vi "DAQ_finite.vi"(8 "error in":errorcluster) -> (0 "error out":errorcluster, 3 "task out":refnum<k21>)   [LabVIEW 2019]
uses:
  <vilib>/DAQmx/create/channels.llb/DAQmx Create Channel (AI-Voltage-Basic).vi
  <vilib>/DAQmx/configure/timing.llb/DAQmx Timing (Sample Clock).vi
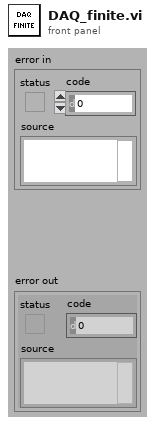
[diagram p1: front panel]
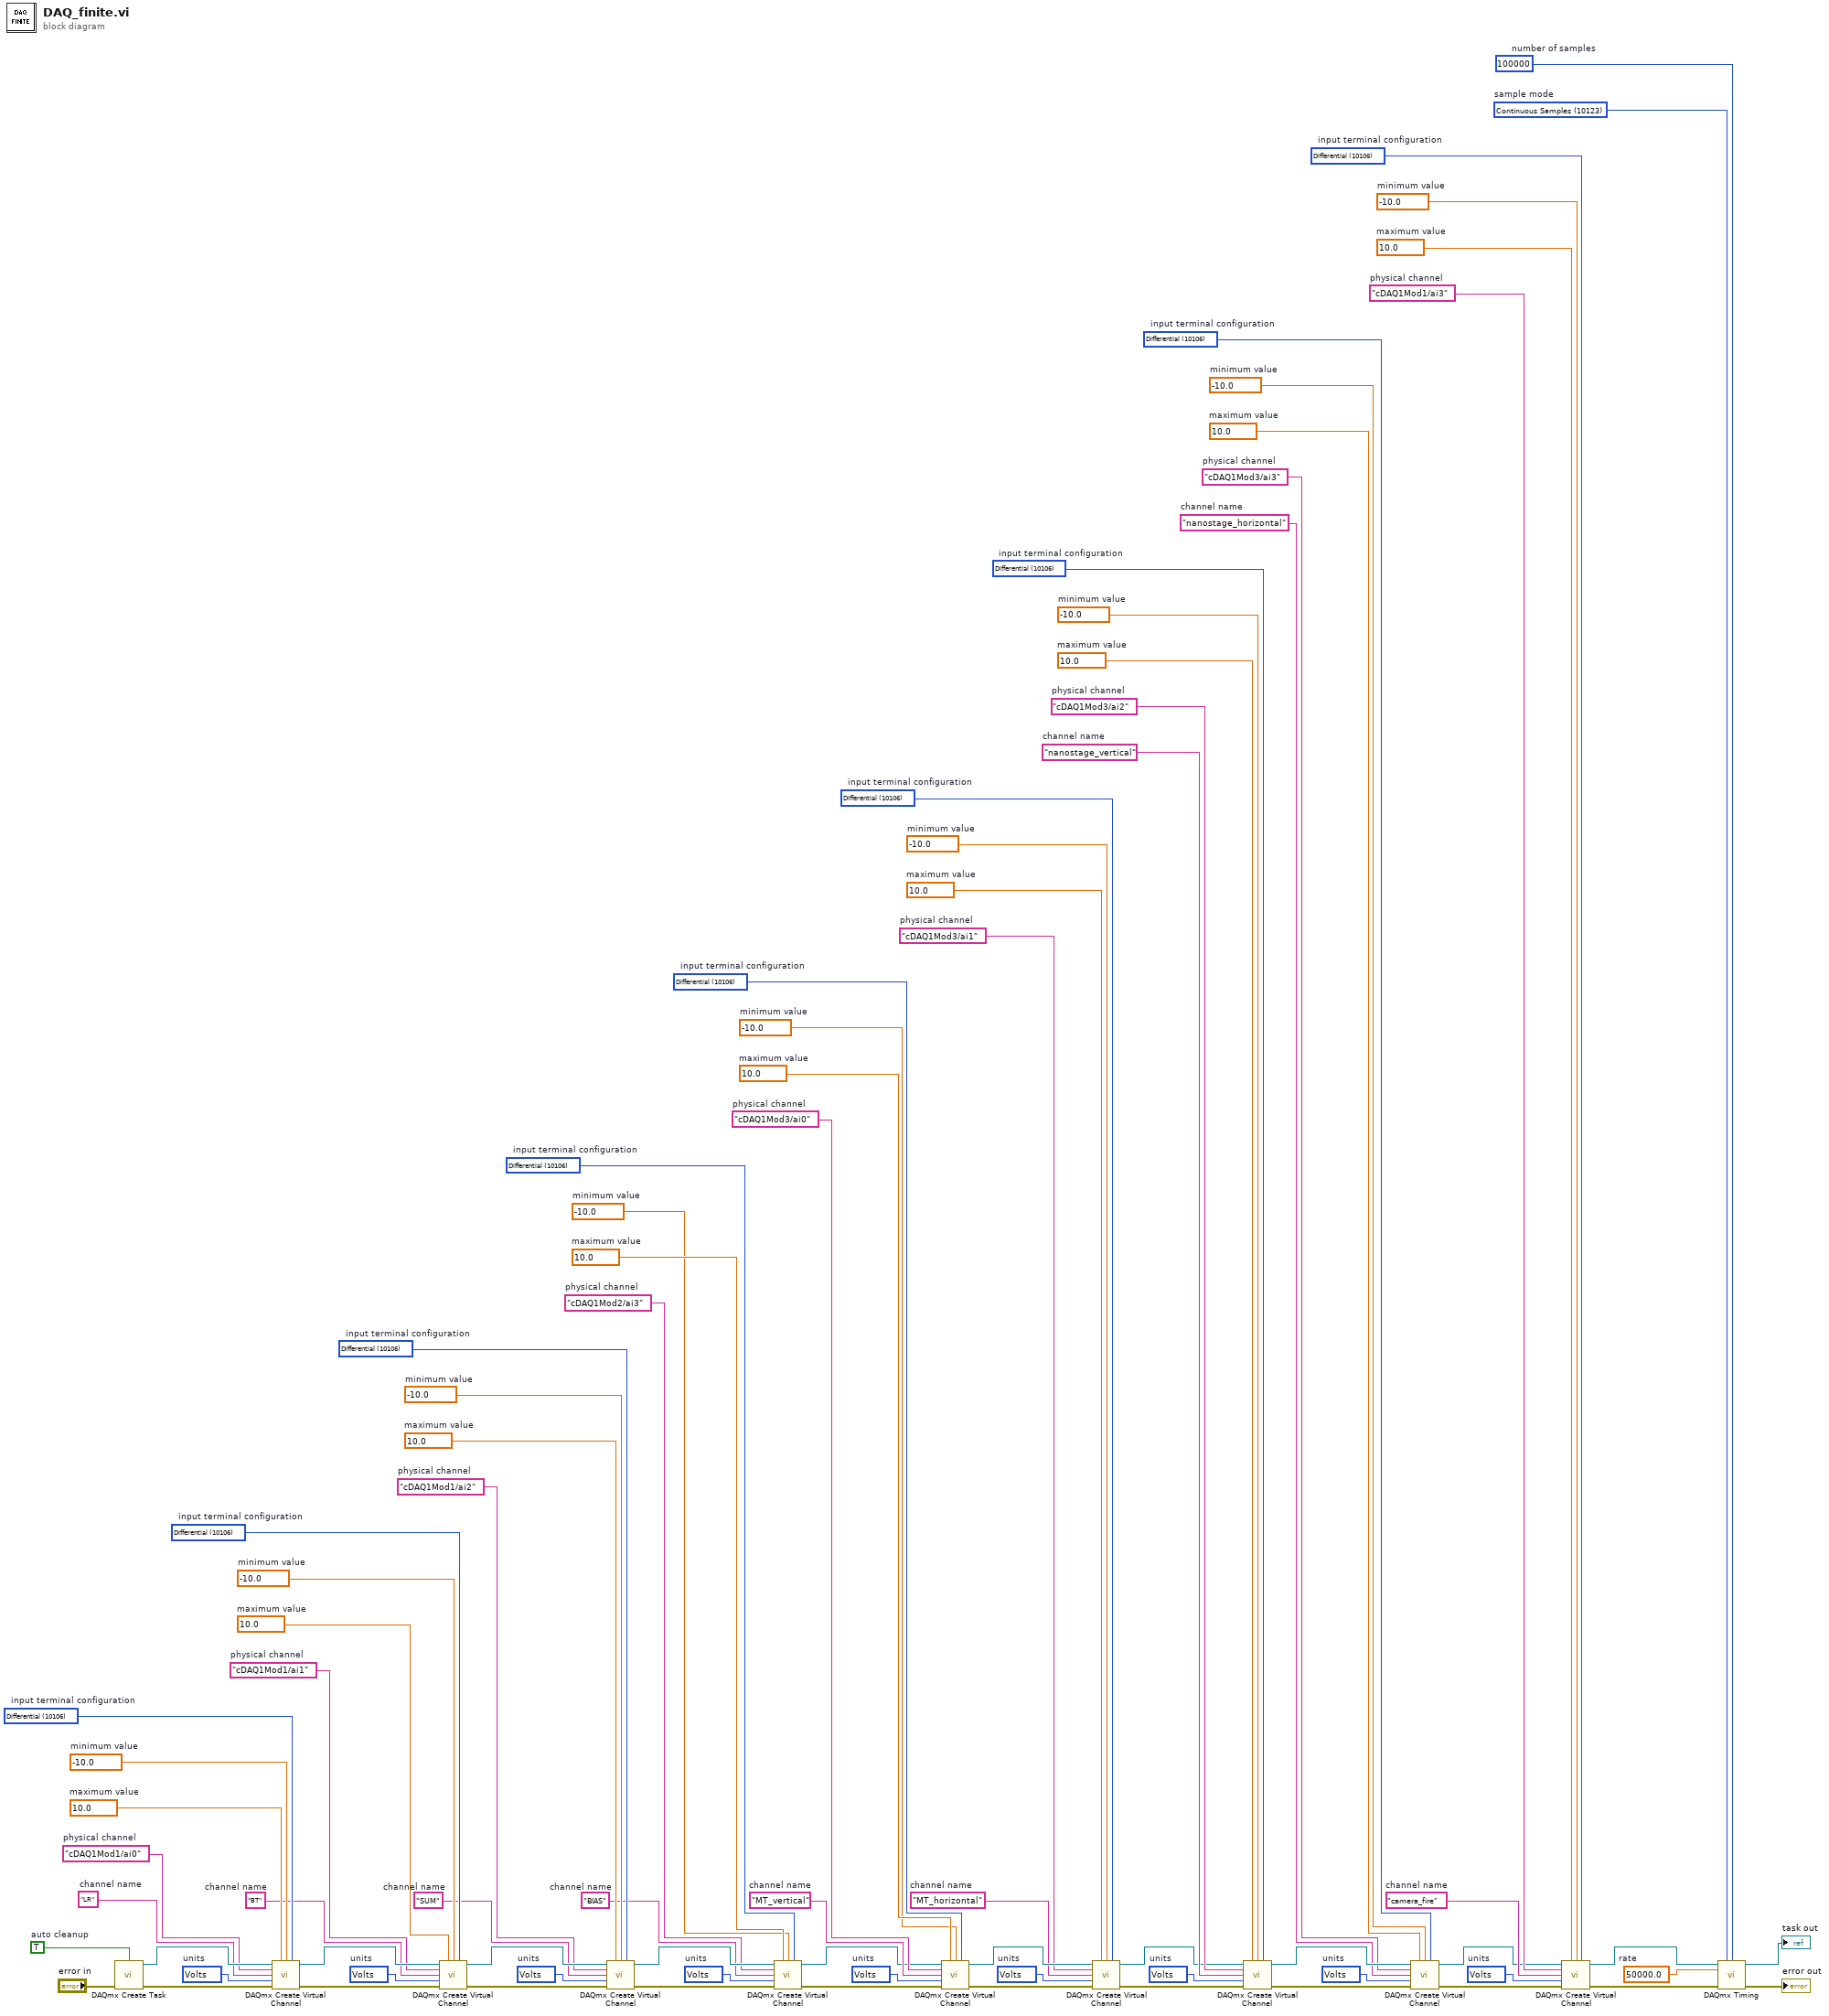
[diagram p0: block diagram]
diagram:
  w3 = 10123 items=["Finite Samples"=10178, "Continuous Samples"=10123, "Hardware Timed Single Point"=12522]  # sample mode
  w4 = 100000  # number of samples
  w5 = 50000.0  # rate
  w10 = 10106 items=["default"=-1, "RSE"=10083, "NRSE"=10078, "Differential"=10106, "Pseudodifferential"=12529]  # input terminal configuration
  w11 = 10348 items=["Volts"=10348, "From Custom Scale"=10065]  # units
  w12 = "camera_fire"  # channel name
  w13 = -10.0  # minimum value
  w14 = 10.0  # maximum value
  w15 = "cDAQ1Mod1/ai3"  # physical channel
  w20 = 10106 items=["default"=-1, "RSE"=10083, "NRSE"=10078, "Differential"=10106, "Pseudodifferential"=12529]  # input terminal configuration
  w21 = 10348 items=["Volts"=10348, "From Custom Scale"=10065]  # units
  w22 = "nanostage_horizontal"  # channel name
  w23 = -10.0  # minimum value
  w24 = 10.0  # maximum value
  w25 = "cDAQ1Mod3/ai3"  # physical channel
  w27 = 10106 items=["default"=-1, "RSE"=10083, "NRSE"=10078, "Differential"=10106, "Pseudodifferential"=12529]  # input terminal configuration
  w28 = 10348 items=["Volts"=10348, "From Custom Scale"=10065]  # units
  w29 = "nanostage_vertical"  # channel name
  w31 = -10.0  # minimum value
  w32 = 10.0  # maximum value
  w33 = "cDAQ1Mod3/ai2"  # physical channel
  w34 = 10106 items=["default"=-1, "RSE"=10083, "NRSE"=10078, "Differential"=10106, "Pseudodifferential"=12529]  # input terminal configuration
  w35 = 10348 items=["Volts"=10348, "From Custom Scale"=10065]  # units
  w36 = "MT_horizontal"  # channel name
  w37 = -10.0  # minimum value
  w38 = 10.0  # maximum value
  w39 = "cDAQ1Mod3/ai1"  # physical channel
  w41 = 10106 items=["default"=-1, "RSE"=10083, "NRSE"=10078, "Differential"=10106, "Pseudodifferential"=12529]  # input terminal configuration
  w42 = 10348 items=["Volts"=10348, "From Custom Scale"=10065]  # units
  w43 = "MT_vertical"  # channel name
  w45 = -10.0  # minimum value
  w46 = 10.0  # maximum value
  w47 = "cDAQ1Mod3/ai0"  # physical channel
  w48 = 10106 items=["default"=-1, "RSE"=10083, "NRSE"=10078, "Differential"=10106, "Pseudodifferential"=12529]  # input terminal configuration
  w49 = 10348 items=["Volts"=10348, "From Custom Scale"=10065]  # units
  w50 = "BIAS"  # channel name
  w51 = -10.0  # minimum value
  w52 = 10.0  # maximum value
  w53 = "cDAQ1Mod2/ai3"  # physical channel
  w55 = 10106 items=["default"=-1, "RSE"=10083, "NRSE"=10078, "Differential"=10106, "Pseudodifferential"=12529]  # input terminal configuration
  w56 = 10348 items=["Volts"=10348, "From Custom Scale"=10065]  # units
  w57 = "SUM"  # channel name
  w59 = -10.0  # minimum value
  w60 = 10.0  # maximum value
  w61 = "cDAQ1Mod1/ai2"  # physical channel
  w63 = 10106 items=["default"=-1, "RSE"=10083, "NRSE"=10078, "Differential"=10106, "Pseudodifferential"=12529]  # input terminal configuration
  w64 = 10348 items=["Volts"=10348, "From Custom Scale"=10065]  # units
  w65 = "BT"  # channel name
  w67 = -10.0  # minimum value
  w68 = 10.0  # maximum value
  w69 = "cDAQ1Mod1/ai1"  # physical channel
  w71 = 10106 items=["default"=-1, "RSE"=10083, "NRSE"=10078, "Differential"=10106, "Pseudodifferential"=12529]  # input terminal configuration
  w72 = 10348 items=["Volts"=10348, "From Custom Scale"=10065]  # units
  w73 = "LR"  # channel name
  w75 = -10.0  # minimum value
  w76 = 10.0  # maximum value
  w77 = "cDAQ1Mod1/ai0"  # physical channel
  w79 = TRUE  # auto cleanup
  n1 = call <vilib>:"DAQmx Create Task.vi"("auto cleanup"=w79, "error in"="error in") -> ("task out"=w78:refnum<k21>, "error out"=w80:errorcluster)  [unwired: 12 in]
  n2 = call-poly <vilib>:"DAQmx Create Virtual Channel.vi"("task in"=w78, "maximum value"=w76, "minimum value"=w75, "input terminal configuration"=w71, "physical channels"=w77, "name to assign"=w73, "units"=w72, "error in"=w80) -> ("task out"=w70:refnum<k21>, "error out"=w74:errorcluster)  [unwired: 6 in]
  n3 = call-poly <vilib>:"DAQmx Create Virtual Channel.vi"("task in"=w70, "maximum value"=w68, "minimum value"=w67, "input terminal configuration"=w63, "physical channels"=w69, "name to assign"=w65, "units"=w64, "error in"=w74) -> ("task out"=w62:refnum<k21>, "error out"=w66:errorcluster)  [unwired: 6 in]
  n4 = call-poly <vilib>:"DAQmx Create Virtual Channel.vi"("task in"=w62, "maximum value"=w60, "minimum value"=w59, "input terminal configuration"=w55, "physical channels"=w61, "name to assign"=w57, "units"=w56, "error in"=w66) -> ("task out"=w54:refnum<k21>, "error out"=w58:errorcluster)  [unwired: 6 in]
  n5 = call-poly <vilib>:"DAQmx Create Virtual Channel.vi"("task in"=w54, "maximum value"=w52, "minimum value"=w51, "input terminal configuration"=w48, "physical channels"=w53, "name to assign"=w50, "units"=w49, "error in"=w58) -> ("task out"=w17:refnum<k21>, "error out"=w16:errorcluster)  [unwired: 6 in]
  n6 = call-poly <vilib>:"DAQmx Create Virtual Channel.vi"("task in"=w17, "maximum value"=w46, "minimum value"=w45, "input terminal configuration"=w41, "physical channels"=w47, "name to assign"=w43, "units"=w42, "error in"=w16) -> ("task out"=w40:refnum<k21>, "error out"=w44:errorcluster)  [unwired: 6 in]
  n7 = call-poly <vilib>:"DAQmx Create Virtual Channel.vi"("task in"=w40, "maximum value"=w38, "minimum value"=w37, "input terminal configuration"=w34, "physical channels"=w39, "name to assign"=w36, "units"=w35, "error in"=w44) -> ("task out"=w19:refnum<k21>, "error out"=w18:errorcluster)  [unwired: 6 in]
  n8 = call-poly <vilib>:"DAQmx Create Virtual Channel.vi"("task in"=w19, "maximum value"=w32, "minimum value"=w31, "input terminal configuration"=w27, "physical channels"=w33, "name to assign"=w29, "units"=w28, "error in"=w18) -> ("task out"=w26:refnum<k21>, "error out"=w30:errorcluster)  [unwired: 6 in]
  n9 = call-poly <vilib>:"DAQmx Create Virtual Channel.vi"("task in"=w26, "maximum value"=w24, "minimum value"=w23, "input terminal configuration"=w20, "physical channels"=w25, "name to assign"=w22, "units"=w21, "error in"=w30) -> ("task out"=w9:refnum<k21>, "error out"=w8:errorcluster)  [unwired: 6 in]
  n10 = call-poly <vilib>:"DAQmx Create Virtual Channel.vi"("task in"=w9, "maximum value"=w14, "minimum value"=w13, "input terminal configuration"=w10, "physical channels"=w15, "name to assign"=w12, "units"=w11, "error in"=w8) -> ("task out"=w2:refnum<k21>, "error out"=w1:errorcluster)  [unwired: 6 in]
  n11 = call-poly <vilib>:"DAQmx Timing.vi"("task/channels in"=w2, "sample mode"=w3, "samples per channel"=w4, "rate"=w5, "error in"=w1) -> ("task out"=→"task out":refnum<k21>, "error out"=→"error out":errorcluster)  [unwired: 9 in]
